vi "manual power set.vi"(7 "DAQ cluster in":T1 {"temp"."utility"."therm volt" format="%_6g"; "temp"."utility"."heat volt in" format="%_6g"; "temp"."utility"."heat volt out" format="%_6g"; "temp"."utility"."power out" format="%_6g"; "temp"."utility"."H Vmax" format="%_6g"; "temp"."T exec"."man power" format="%_6g"; "temp"."T exec"."exec setpoint" format="%_6g"; "temp"."T params"."Settle Time" step=1.0; "temp"."T params"."Settle Bandwidth" step=0.01; "temp"."T params"."Derivative Tme" step=0.01; "temp"."T params"."Integral Time" step=1.0; "temp"."T params"."Control Bandwidth" step=0.1; "temp"."T params"."Setpoint" step=0.1; "temp"."T status"."Setpoint" format="%_6g"; "temp"."T status"."Power" format="%_6g"; "temp"."T status"."Temp" format="%_6g"}) -> (8 "DAQ cluster out":T1 {"temp"."utility"."therm volt" format="%_6g"; "temp"."utility"."heat volt in" format="%_6g"; "temp"."utility"."heat volt out" format="%_6g"; "temp"."utility"."power out" format="%_6g"; "temp"."utility"."H Vmax" format="%_6g"; "temp"."T exec"."man power" format="%_6g"; "temp"."T exec"."exec setpoint" format="%_6g"; "temp"."T params"."Settle Time" step=1.0; "temp"."T params"."Settle Bandwidth" step=0.01; "temp"."T params"."Derivative Tme" step=0.01; "temp"."T params"."Integral Time" step=1.0; "temp"."T params"."Control Bandwidth" step=0.1; "temp"."T params"."Setpoint" step=0.1; "temp"."T status"."Setpoint" format="%_6g"; "temp"."T status"."Power" format="%_6g"; "temp"."T status"."Temp" format="%_6g"})   [LabVIEW 2019]
doc: "This subVI is one of the states of the DAQ state machine in the bug experiment.\n\nThis state sets the user selected manual power.\n\nIt proceeds to output power next.\n\nPaul K Dixon\nP3600\nCSUSB Physics"
uses:
  typedefs/DAQ state cluster.ctl
  typedefs/DAQ state enum.ctl
  typedefs/temp cont cluster.ctl
  typedefs/temp exec cluster.ctl
  typedefs/temp mode enum.ctl
  typedefs/temp indicator.ctl
  typedefs/temp control status.ctl
  typedefs/PID control parameters.ctl
  typedefs/temp cont utility.ctl
  typedefs/measurement.ctl
  typedefs/wvfm acq params.ctl
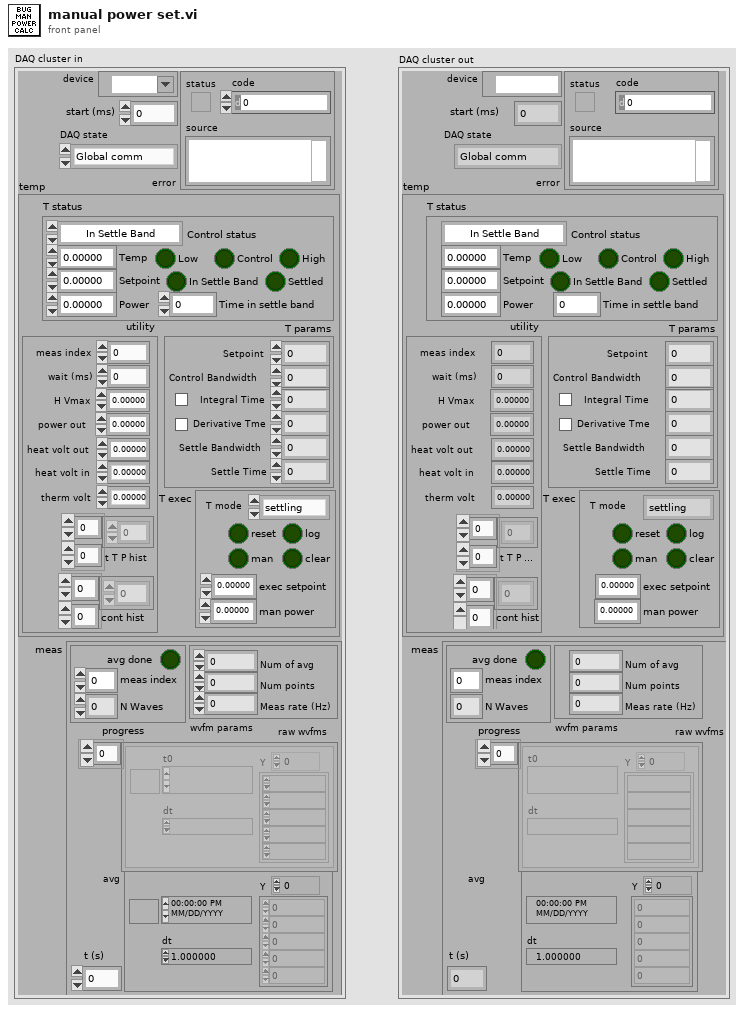
[diagram p1: front panel]
types:
  T1 = typedef "DAQ state cluster.ctl" = cluster{"DAQ state":T2, "temp":T3, "meas":T10, "device":tag, "error":errorcluster, "start (ms)":i32}
  T2 = typedef "DAQ state enum.ctl" = enum16{"Global comm", "Meas T & P", "PID power calc", "Man Power set", "Output Power", "Wait", "Meas wvfm", "Avg wvfm", "Exit"}
  T3 = typedef "temp cont cluster.ctl" = cluster{"T exec":T4, "T status":T6, "T params":T8, "utility":T9}
  T4 = typedef "temp exec cluster.ctl" = cluster{"T mode":T5, "exec setpoint":dbl, "reset":bool, "man power":dbl, "man":bool, "log":bool, "clear":bool}
  T5 = typedef "temp mode enum.ctl" = enum16{"settling", "measuring", "holding", "Exit"}
  T6 = typedef "temp indicator.ctl" = cluster{"Control status":T7, "Temp":dbl, "Power":dbl, "Time in settle band":dbl, "Settled":bool, "Low":bool, "High":bool, "Setpoint":dbl, "Control":bool, "In Settle Band":bool}
  T7 = typedef "temp control status.ctl" = enum16{"In Settle Band", "In Control Band", "Below Control Band", "Above Control Band"}
  T8 = typedef "PID control parameters.ctl" = cluster{"Setpoint":dbl, "Control Bandwidth":dbl, "Integral Time":dbl, "Int\nON":bool, "Derivative Tme":dbl, "Der\nON":bool, "Settle Bandwidth":dbl, "Settle Time":dbl}
  T9 = typedef "temp cont utility.ctl" = cluster{"meas index":i32, "wait (ms)":i32, "H Vmax":dbl, "power out":dbl, "heat volt out":dbl, "heat volt in":dbl, "therm volt":dbl, "t T P hist":dbl[][], "cont hist":dbl[][]}
  T10 = typedef "measurement.ctl" = cluster{"wvfm params":T11, "avg":waveform(dbl), "raw wvfms":waveform(dbl)[], "progress":cluster{"avg done":bool, "meas index":i32, "N waves":i32}, "t (s)":dbl}
  T11 = typedef "wvfm acq params.ctl" = cluster{"Num of avg":i32, "Num points":i32, "Meas rate (Hz)":dbl}
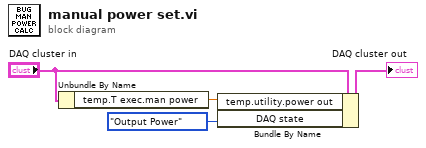
[diagram p0: block diagram]
diagram:
  n1 = Unbundle By Name("DAQ cluster in") -> ("temp.T exec.man power"=w2:dbl)
  n2 = Bundle By Name(cluster="DAQ cluster in", "temp.utility.power out"=w2, "DAQ state"=DAQ_state_enum."Output Power") -> (→"DAQ cluster out":T1)
